vi "校准记录.vi"(8 "error in (no error)":errorcluster, 9 "曲线模型":T1={"标液浓度1"=0.0, "测量吸光度1"=0.0, "样品1启用"=FALSE, "标液浓度2"=0.0, "测量吸光度2"=0.0, "样品2启用"=FALSE, "标液浓度3"=0.0, "测量吸光度3"=0.0, "样品3启用"=FALSE, "标液浓度4"=0.0, "测量吸光度4"=0.0, "样品4启用"=FALSE, "标液浓度5"=0.0, "测量吸光度5"=0.0, "样品5启用"=FALSE, "模型"=enum."线性", "精度"=4.0, "XY图"=[], "拟合公式"="", "r^2"=0.0, "标样一校准时间"=timestamp(0 s since 1904-01-01), "标样二校准时间"=timestamp(0 s since 1904-01-01), "标样三校准时间"=timestamp(0 s since 1904-01-01), "标样四校准时间"=timestamp(0 s since 1904-01-01), "标样五校准时间"=timestamp(0 s since 1904-01-01), "二次方程"={"c"=0.0, "x"=0.0, "x^2"=0.0}, "标定时间"=timestamp(0 s since 1904-01-01), "拟合公式 2"="", "r^2 2"=0.0} {"r^2 2" format="%.7f"; "标定时间" format="%<%m/%d/%y %H:%M:%S>T"; "标样五校准时间" format="%<%m/%d/%y %H:%M:%S>T"; "标样四校准时间" format="%<%m/%d/%y %H:%M:%S>T"; "标样三校准时间" format="%<%m/%d/%y %H:%M:%S>T"; "标样二校准时间" format="%<%m/%d/%y %H:%M:%S>T"; "标样一校准时间" format="%<%m/%d/%y %H:%M:%S>T"; "r^2" format="%.7f"; "测量吸光度5" format="%#.6f"; "测量吸光度4" format="%#.6f"; "测量吸光度3" format="%#.6f"; "测量吸光度2" format="%#.6f"; "测量吸光度1" format="%#.6f"}, 10 "量程":enum16{"低量程", "高量程"}(ring), 11 "测量模式":string="所有测量模式") -> (0 "error out":errorcluster)   [LabVIEW 2016, in "斯坦道CODMn新电路板.lvlib"]
panel:
  out "结果字符串":string
  in  "data in":T2
  # "校准时间"
  # "标液浓度"
  # "吸光值显示"
  # "标液一"
  # "标液二"
  # "标液三"
  # "零点"
  # "跨度"
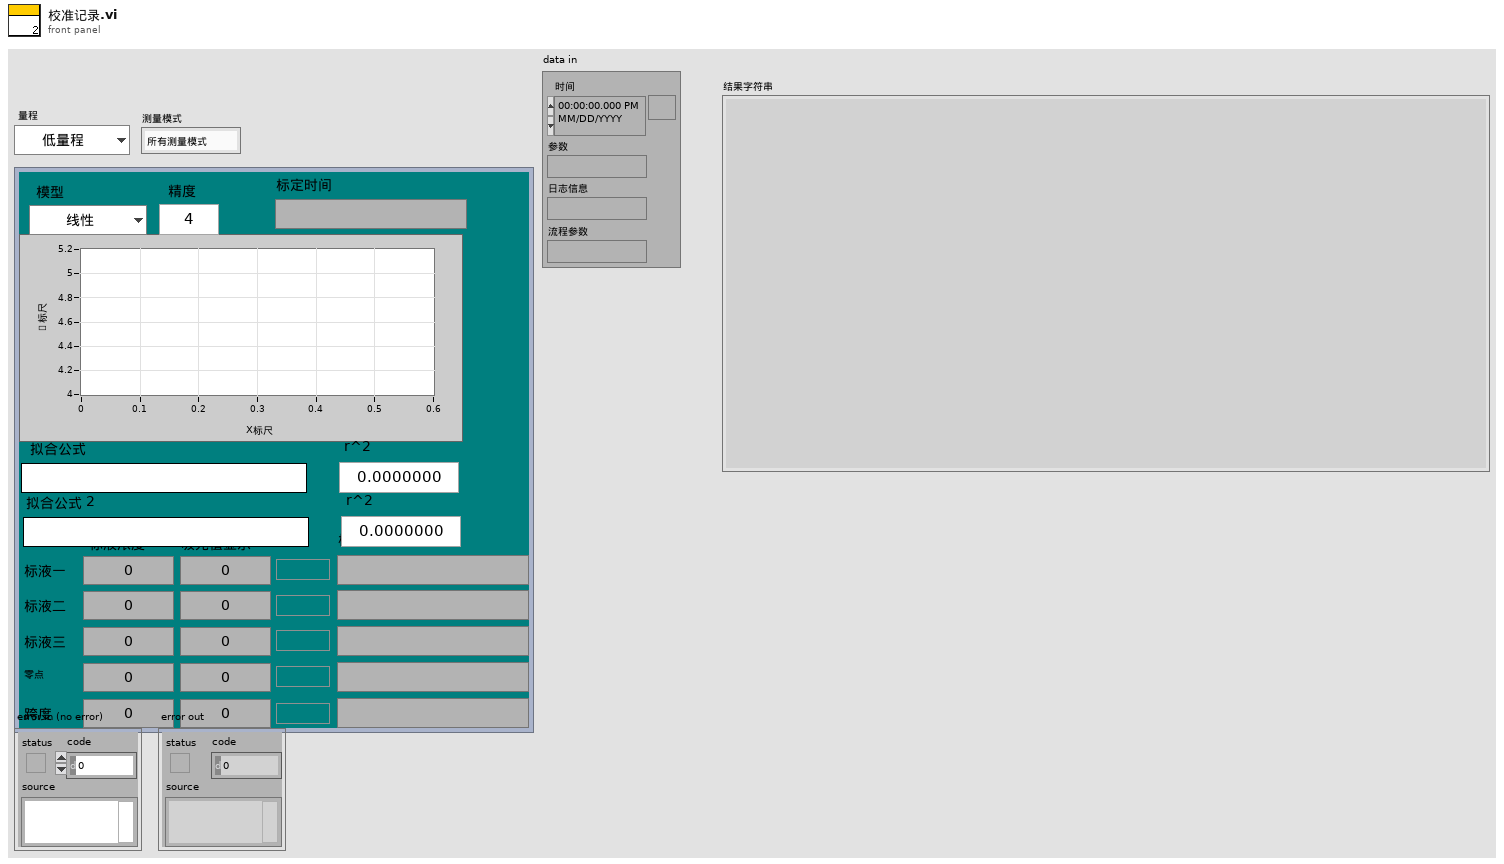
[diagram p1: front panel]
types:
  T1 = cluster{"标液浓度1":dbl, "测量吸光度1":dbl, "样品1启用":bool, "标液浓度2":dbl, "测量吸光度2":dbl, "样品2启用":bool, "标液浓度3":dbl, "测量吸光度3":dbl, "样品3启用":bool, "标液浓度4":dbl, "测量吸光度4":dbl, "样品4启用":bool, "标液浓度5":dbl, "测量吸光度5":dbl, "样品5启用":bool, "模型":enum32{"线性", "多项式", "折线"}, "精度":dbl, "XY图":cluster{"X Values":dbl[], "Y Values":dbl[]}[], "拟合公式":string, "r^2":dbl, "标样一校准时间":timestamp, "标样二校准时间":timestamp, "标样三校准时间":timestamp, "标样四校准时间":timestamp, "标样五校准时间":timestamp, "二次方程":cluster{"c":dbl, "x":dbl, "x^2":dbl}, "标定时间":timestamp, "拟合公式 2":string, "r^2 2":dbl}
  T2 = cluster{"时间":timestamp, "参数":string, "日志信息":string, "流程参数":string}
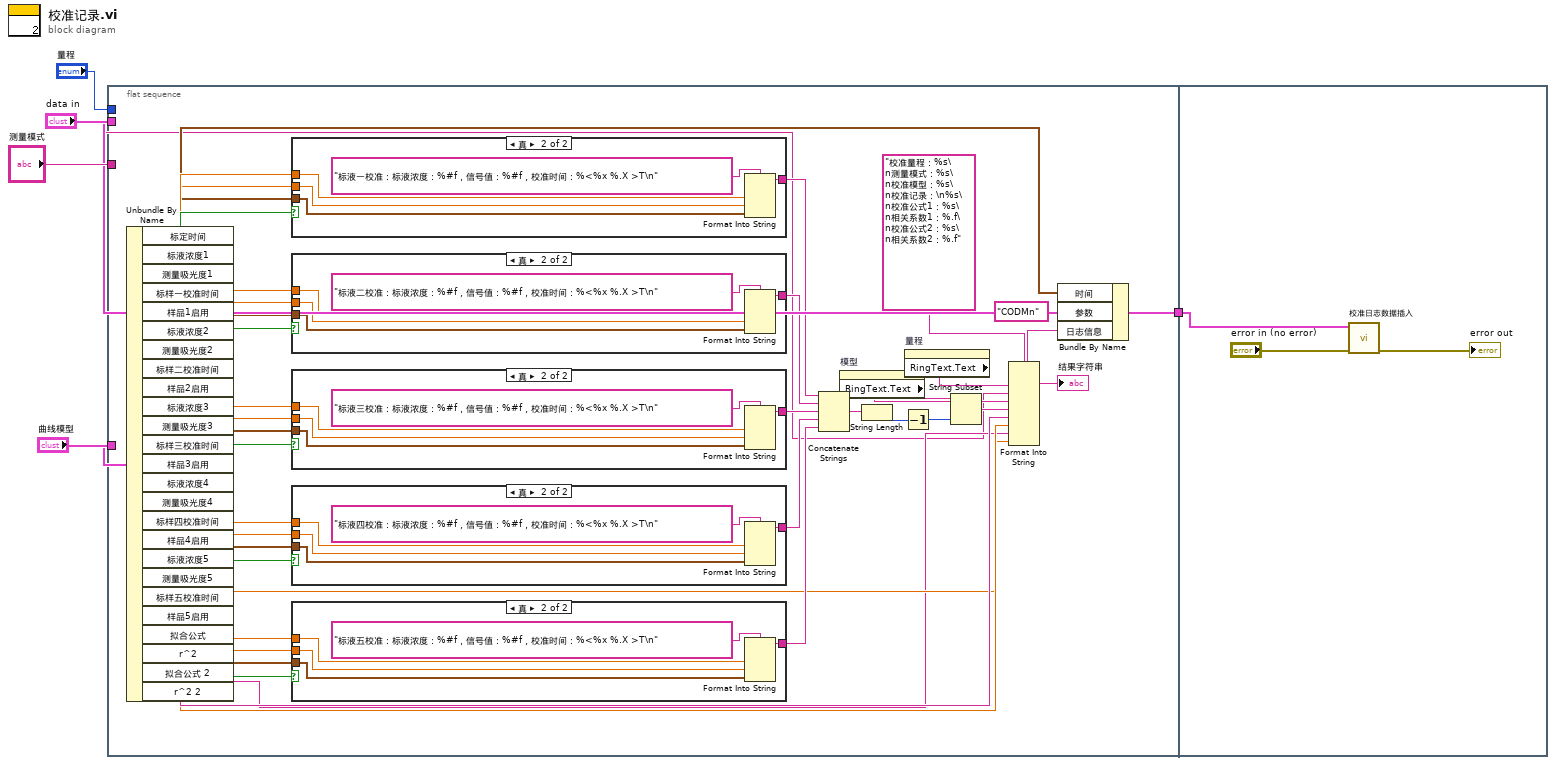
[diagram p0: block diagram]
diagram:
  n1 = flat-sequence {
    tunnel: "量程" -> [_]
    tunnel: "曲线模型" -> [w44]
    tunnel: "data in" -> [w48]
    tunnel: [w47] -> w2
    tunnel: "测量模式" -> [w6]
    tunnel: w2 -> [w74]
    frame #0 {
      n2 = Unbundle By Name(w44) -> ("标定时间"=w12:timestamp, "标液浓度1"=w42:dbl, "测量吸光度1"=w41:dbl, "标样一校准时间"=w40:timestamp, "样品1启用"=w43:bool, "标液浓度2"=w39:dbl, "测量吸光度2"=w38:dbl, "标样二校准时间"=w37:timestamp, "样品2启用"=w36:bool, "标液浓度3"=w35:dbl, "测量吸光度3"=w34:dbl, "标样三校准时间"=w33:timestamp, "样品3启用"=w32:bool, "标液浓度4"=w31:dbl, "测量吸光度4"=w30:dbl, "标样四校准时间"=w29:timestamp, "样品4启用"=w28:bool, "标液浓度5"=w27:dbl, "测量吸光度5"=w26:dbl, "标样五校准时间"=w25:timestamp, "样品5启用"=w24:bool, "拟合公式"=w18:string, "r^2"=w17:dbl, "拟合公式 2"=w10:string, "r^2 2"=w11:dbl)
      n3 = case shown="真" w43 {
        tunnel: w42 -> [_ w72]
        tunnel: w41 -> [_ w71]
        tunnel: w40 -> [_ w70]
        tunnel: [_ w69] -> w23
        frame False {
        }
        frame True {
          n4 = Format Into String(format string="标液一校准：标液浓度：%#f，信号值：%#f，校准时间：%<%x %.X >T\n" ("格式字符串"), w72, w71, w70) -> (resulting string=w69:string)  [unwired: 2 in, 1 out]
        }
      }
      n5 = case shown="真" w36 {
        tunnel: w39 -> [_ w67]
        tunnel: w38 -> [_ w66]
        tunnel: w37 -> [_ w65]
        tunnel: [_ w64] -> w22
        frame False {
        }
        frame True {
          n6 = Format Into String(format string="标液二校准：标液浓度：%#f，信号值：%#f，校准时间：%<%x %.X >T\n" ("格式字符串"), w67, w66, w65) -> (resulting string=w64:string)  [unwired: 2 in, 1 out]
        }
      }
      n7 = case shown="真" w32 {
        tunnel: w35 -> [_ w62]
        tunnel: w34 -> [_ w61]
        tunnel: w33 -> [_ w60]
        tunnel: [_ w59] -> w21
        frame False {
        }
        frame True {
          n8 = Format Into String(format string="标液三校准：标液浓度：%#f，信号值：%#f，校准时间：%<%x %.X >T\n" ("格式字符串"), w62, w61, w60) -> (resulting string=w59:string)  [unwired: 2 in, 1 out]
        }
      }
      n9 = case shown="真" w28 {
        tunnel: w31 -> [_ w57]
        tunnel: w30 -> [_ w56]
        tunnel: w29 -> [_ w55]
        tunnel: [_ w54] -> w20
        frame False {
        }
        frame True {
          n10 = Format Into String(format string="标液四校准：标液浓度：%#f，信号值：%#f，校准时间：%<%x %.X >T\n" ("格式字符串"), w57, w56, w55) -> (resulting string=w54:string)  [unwired: 2 in, 1 out]
        }
      }
      n11 = case shown="真" w24 {
        tunnel: w27 -> [_ w52]
        tunnel: w26 -> [_ w51]
        tunnel: w25 -> [_ w50]
        tunnel: [_ w49] -> w19
        frame False {
        }
        frame True {
          n12 = Format Into String(format string="标液五校准：标液浓度：%#f，信号值：%#f，校准时间：%<%x %.X >T\n" ("格式字符串"), w52, w51, w50) -> (resulting string=w49:string)  [unwired: 2 in, 1 out]
        }
      }
      n13 = Concatenate Strings(w23, w22, w21, w20, w19) -> (w15:string)
      n14 = property on="模型" class="Enum (严格)"() -> ("RingText.Text"=w9:string)  [unwired: 2 in, 2 out]
      n15 = String Length(string=w15) -> (length=w14:i32)
      n16 = Decrement(x=w14) -> (x-1=w13:i32)
      n17 = property on="量程" class="Enum (严格)"() -> ("RingText.Text"=w7:string)  [unwired: 2 in, 2 out]
      n18 = String Subset(string=w15, length (rest)=w13) -> (substring=w16:string)  [unwired: 1 in]
      n19 = Format Into String(format string="校准量程：%s\n测量模式：%s\n校准模型：%s\n校准记录：\n%s\n校准公式1：%s\n相关系数1：%.f\n校准公式2：%s\n相关系数2：%.f" ("格式字符串"), w7, w6, w9, w16, w18, w17, w10, w11) -> (resulting string=w46:string)  [unwired: 2 in, 1 out]
      "结果字符串" <- w46
      n20 = Bundle By Name(cluster=w48, "时间"=w12, "参数"="CODMn", "日志信息"=w46) -> (w47:T2)
    }
    frame #1 {
      n21 = call "校准日志数据插入.vi"("data"=w74, "错误输入（无错误）"="error in (no error)") -> ("错误输出"=→"error out":errorcluster)  [unwired: 8 in]
    }
  }
